vi "_RT_CtrlLoop_Pub_Get_Address.vi"(9 "Response Str":string="@253AcK253;FF") -> (2 "Is Exist?":bool, 3 "Address Str":string)   [LabVIEW 2018]
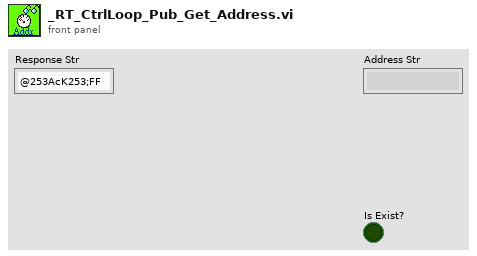
[diagram p1: front panel]
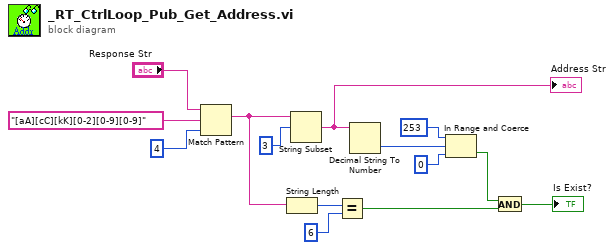
[diagram p0: block diagram]
diagram:
  n1 = Match Pattern(string="Response Str", regular expression="[aA][cC][kK][0-2][0-9][0-9]", offset (0)=4) -> (match substring=w10:string)  [unwired: 3 out]
  n2 = String Length(string=w10) -> (length=w13:i32)
  n3 = String Subset(string=w10, offset (0)=3) -> (substring=w5:string)  [unwired: 1 in]
  "Address Str" <- w5
  n4 = Equal?(x=w13, y=6) -> (x = y?=w3:bool)
  n5 = Decimal String To Number(string=w5) -> (number=w8:i32)  [unwired: 2 in, 1 out]
  n6 = In Range and Coerce(upper limit=253, x=w8, lower limit=0) -> (In Range?=w4:bool)  [unwired: 1 out]
  n7 = And(x=w4, y=w3) -> (x .and. y?=→"Is Exist?":bool)
